vi "Query Max Current Limit.vi"(8 "error in (no error)":errorcluster, 9 "voltage level (0.0 Volts)":dbl[unit] format="%^.2e", 10 "channel name (\"CHANNEL1\")":string="CHANNEL1", 11 "CS++DCPwr in":refnum<class "CS++DCPwr.lvclass">) -> (0 "error out":errorcluster, 2 "max current limit":dbl[unit] format="%^.2e", 3 "CS++DCPwr out":refnum<class "CS++DCPwr.lvclass">)   [LabVIEW 2013, in "CS++DCPwr.lvlib" / "CS++DCPwr.lvclass"]
doc: "This VI returns the maximum programmable current limit that the power supply accepts for a particular voltage level on a channel for the output range to which the power supply is currently configured."
uses:
  CS++DCPwr.lvclass
  CSPP_Core/Classes/CS++ProcessVariables/ProcessVariable/PV.lvclass
  CSPP_Core/Classes/CS++ProcessVariables/ProcessVariable/PV.lvclass/PV.ctl
  CS++DCPwr.lvclass/CS++DCPwr.ctl
  CSPP_Core/Classes/CS++ProcessVariables/PVConnection/PVConnection.lvclass
  CSPP_Core/Classes/CS++ProcessVariables/ProcessVariable/Write Data.vi
  CSPP_Core/Classes/CS++ProcessVariables/ProcessVariable/Write Timestamp.vi
  CSPP_Core/Classes/CS++ProcessVariables/ProcessVariable/Write Quality.vi
  CSPP_Core/Classes/CS++ProcessVariables/ProcessVariable/Write status.vi
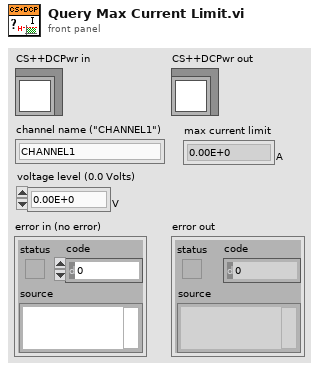
[diagram p1: front panel]
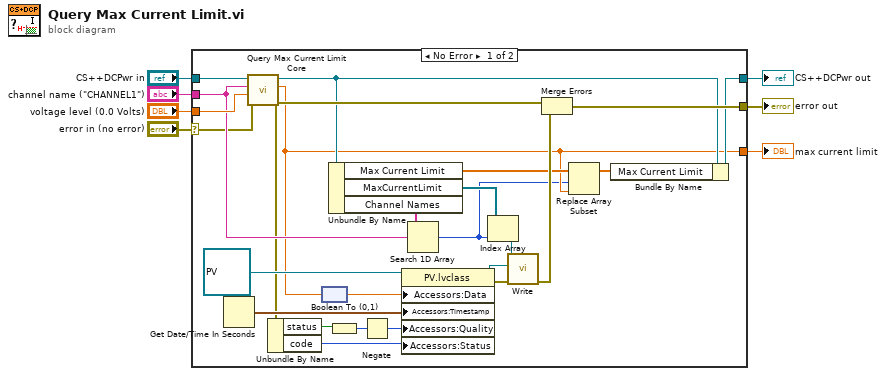
[diagram p0: block diagram]
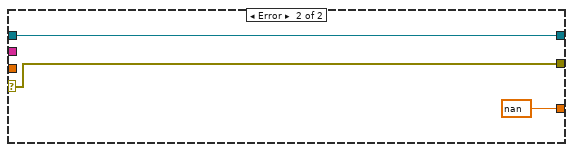
[diagram p2: hidden frame]
diagram:
  n1 = case shown="No Error" "error in (no error)" {
    selector: "error in (no error)" -> [w9 w34]
    tunnel: "CS++DCPwr in" -> [w32 w35]
    tunnel: "voltage level (0.0 Volts)" -> [w31 _]
    tunnel: "channel name (\"CHANNEL1\")" -> [w18 _]
    tunnel: [w16 w34] -> w4
    tunnel: [w14 w35] -> w3
    tunnel: [w11 dbl[unit] nan ("max current limit")] -> w2
    frame No Error {
      n2 = Get Date/Time In Seconds() -> (seconds since 1Jan1904=w30:timestamp)
      n3 = call-dynamic "Query Max Current Limit Core.vi"("error in (no error)"=w9, "voltage level (0.0 Volts)"=w31, "channel name (\"CHANNEL1\")"=w18, "CS++DCPwr in"=w32) -> ("error out"=w17:errorcluster, "max current limit"=w11:dbl[unit], "CS++DCPwr out"=w15:refnum<class "CS++DCPwr.lvclass">)  [unwired: 5 in]
      n4 = Unbundle By Name(w17) -> ("status"=w22:bool, "code"=w20:i32)
      n5 = node(w11) -> (w8:dbl)
      n6 = Unbundle By Name(w15) -> ("Max Current Limit"=w13:dbl[unit][], "MaxCurrentLimit"=w25:refnum<class "PVConnection.lvclass">[], "Channel Names"=w26:string[])
      n7 = Boolean To (0,1)(Boolean=w22) -> (0, 1=w21:i16)
      n8 = Negate(x=w21) -> (-x=w19:i16)
      n9 = property class="PV.lvclass"(reference=refnum<class "PV.lvclass"> refnum ("PV"), "Accessors:Data"=w8, "Accessors:Timestamp"=w30, "Accessors:Quality"=w19, "Accessors:Status"=w20) -> (reference out=w27:refnum<class "PV.lvclass">, error out=w28:errorcluster)  [unwired: 1 in]
      n10 = Search 1D Array(1D array=w26, element=w18) -> (index of element=w10:i32)  [unwired: 1 in]
      n11 = Index Array(array=w25, index=w10) -> (element=w24:refnum<class "PVConnection.lvclass">)
      n12 = call-dynamic "Write.vi"("error in (no error)"=w28, "PV"=w27, "PVConnection in"=w24) -> ("error out"=w23:errorcluster)  [unwired: 7 in, 1 out]
      n13 = Merge Errors(w17, w23) -> (w16:errorcluster)
      n14 = Replace Array Subset(array=w13, new element=w11, index=w10) -> (w12:dbl[unit][])
      n15 = Bundle By Name(cluster=w15, "Max Current Limit"=w12) -> (w14:refnum<class "CS++DCPwr.lvclass">)
    }
    frame Error {
    }
  }
  "error out" <- w4
  "CS++DCPwr out" <- w3
  "max current limit" <- w2
